vi "CreateFileDirectory.vi"(10 "directory":path, 11 "filename":path) -> (3 "filename (copy)":path)   [LabVIEW 2011]
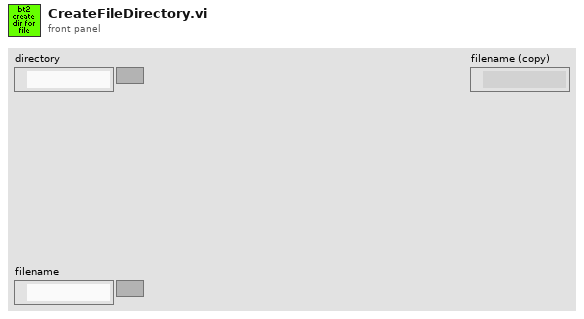
[diagram p1: front panel]
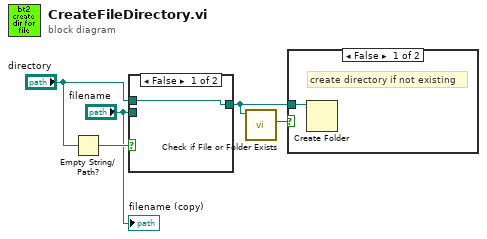
[diagram p0: block diagram]
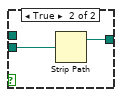
[diagram p2: hidden frame]
diagram:
  n1 = Empty String/Path?(string/path="directory") -> (empty?=w4:bool)
  n2 = case shown="False" w4 {
    tunnel: [w6 w7] -> w2
    tunnel: "filename" -> [_ w8]
    tunnel: "directory" -> [w6 _]
    frame False {
    }
    frame True {
      n3 = Strip Path(path=w8) -> (stripped path=w7:path)  [unwired: 1 out]
    }
  }
  n4 = call <vilib>:"Check if File or Folder Exists.vi"("path"=w2) -> ("file or folder exists?"=w5:bool)  [unwired: 8 in, 2 out]
  n5 = case shown="False" w5 {
    tunnel: w2 -> [w9 _]
    frame False {
      # "create directory if not existing"
      n6 = Create Folder(path (use dialog)=w9) -> ()  [unwired: 2 in, 3 out]
    }
    frame True {
    }
  }
  "filename (copy)" <- "filename"
